vi "niRFUtil MT UTIL Map Bits to Integer Symbols.vi"(0 "input bit stream":i8[](array[numeric]), 5 "bits per integer symbol":i32=1, 7 "bit order":enum16{"MSB first", "LSB first"}(ring), 9 "integer format":enum16{"Unsigned", "Signed"}(ring), 11 "error in (no error)":errorcluster) -> (4 "output integer symbols":i32[](array[numeric]), 15 "error out":errorcluster)   [LabVIEW 2015, in "niRFUtil.lvlib"]
uses:
  niRFUtil.lvlib
  niRFDMT.dll
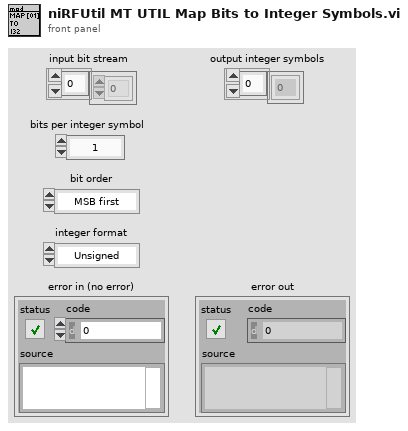
[diagram p1: front panel]
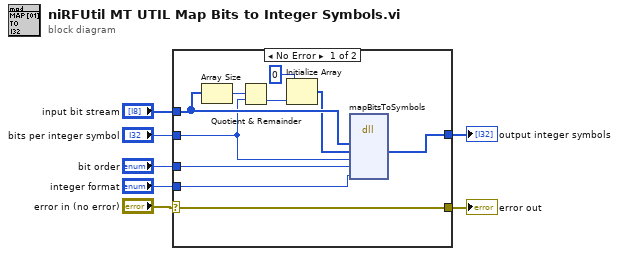
[diagram p0: block diagram]
diagram:
  n1 = case shown="No Error" "error in (no error)" {
    selector: "error in (no error)" -> [w8 w18]
    tunnel: "input bit stream" -> [w16 _]
    tunnel: "bits per integer symbol" -> [w14 _]
    tunnel: [w8 w18] -> w4
    tunnel: "bit order" -> [w17 _]
    tunnel: [w10 _] -> w2
    tunnel: "integer format" -> [w9 _]
    frame No Error {
      n2 = Array Size(array=w16) -> (size(s)=w15:i32)
      n3 = Quotient & Remainder(x=w15, y=w14) -> (floor(x/y)=w13:i32)  [unwired: 1 out]
      n4 = Initialize Array(0, w13) -> (w11:i32[])
      n5 = dll-call lib="C:/Perforce/semoore-sales/Customers/NATI-3813/Noise Floor/LV Filters/ParallelComplexFilterRFUtil/niRFUtil/MT/Utilities/niRFDMT.*" fn="mapBitsToSymbols"("bits"=w16, "symbols"=w11, "bitsPerSymbol"=w14, "bitOrder"=w17, "integer format"=w9) -> ("symbols"=w10:i32[])  [unwired: 5 in, 5 out]
    }
    frame Error {
    }
  }
  "error out" <- w4
  "output integer symbols" <- w2
